vi "WriteToBaseConfigVariant.vi"(6 "Measurement RefreshTime (ms)":u32, 8 "error in (no error)":errorcluster, 9 "Meas":variant, 10 "Config":variant, 11 "NHRGridSim in":refnum<class "NHRGridSim.lvclass">) -> (0 "error out":errorcluster, 3 "NHRGridSim out":refnum<class "NHRGridSim.lvclass">)   [LabVIEW 2018, in "AcPwrPlugins.lvlib" / "NHRGridSim.lvclass"]
uses:
  NHRGridSim.lvclass
  C:/Users/ico/Documents/Projects/NistPluggableModules/AcPwr/AcPwrPlugins/AcPwrBaseClass/AcPwrBase.lvclass
  AcPwrBaseClass/AcPwrBase.lvclass/AcPwrBase.ctl
  AcPwrBaseClass/Accessors/Read BaseConfig.vi
  AcPwrBaseClass/Accessors/Write BaseConfig.vi
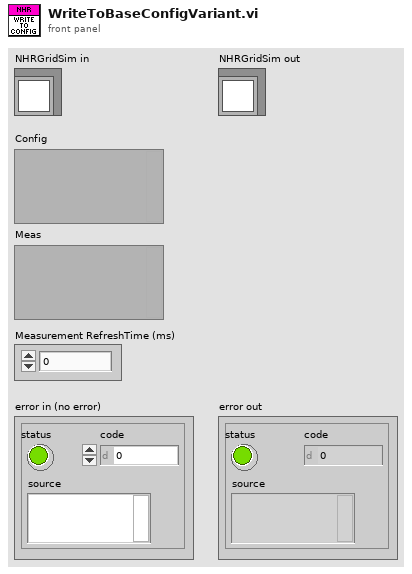
[diagram p1: front panel]
types:
  T1 = typedef "AcPwrPlugins.lvlib/AcPwrBase.lvclass/BaseConfig.ctl" = cluster{"Frequency":dbl, "FrequencyRange":dbl[], "Phases":T2[], "Name":string, "PluginConfigVariant":variant, "PluginMeasVariant":variant}
  T2 = typedef "AcPwrPlugins.lvlib/AcPwrBase.lvclass/Phase.ctl" = cluster{"Name":string, "Enabled":bool, "VoltageLevel":dbl, "Handle":string, "VoltageRange":dbl[], "Connected":bool, "CurrentLimit":dbl, "Waveform":string}
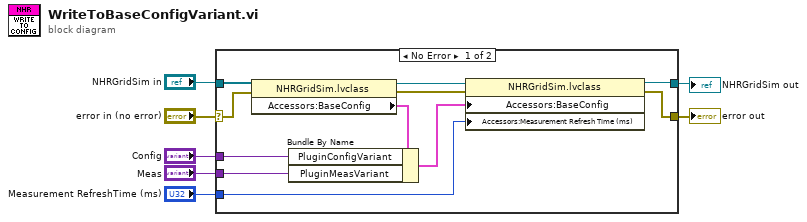
[diagram p0: block diagram]
diagram:
  n1 = case shown="No Error" "error in (no error)" {
    selector: "error in (no error)" -> [w17 w20]
    tunnel: [w13 w20] -> w5
    tunnel: [w11 w19] -> w6
    tunnel: "NHRGridSim in" -> [w18 w19]
    tunnel: "Config" -> [w14 _]
    tunnel: "Meas" -> [w9 _]
    tunnel: "Measurement RefreshTime (ms)" -> [w8 _]
    frame No Error {
      n2 = property class="NHRGridSim.lvclass"(reference=w18, error in=w17) -> (reference out=w12:refnum<class "NHRGridSim.lvclass">, error out=w16:errorcluster, "Accessors:BaseConfig"=w15:T1)
      n3 = Bundle By Name(cluster=w15, "PluginConfigVariant"=w14, "PluginMeasVariant"=w9) -> (w10:T1)
      n4 = property class="NHRGridSim.lvclass"(reference=w12, error in=w16, "Accessors:BaseConfig"=w10, "Accessors:Measurement Refresh Time (ms)"=w8) -> (reference out=w11:refnum<class "NHRGridSim.lvclass">, error out=w13:errorcluster)
    }
    frame Error {
    }
  }
  "error out" <- w5
  "NHRGridSim out" <- w6
